vi "Test Autophase.vi"(8 "error in (no error)":errorcluster, 11 "SR7270 Drivers in":refnum<class "SR7270 Drivers.lvclass">) -> (0 "error out":errorcluster, 3 "SR7270 Drivers out":refnum<class "SR7270 Drivers.lvclass">)   [LabVIEW 2016, in "SR7270 Drivers.lvlib"]
uses:
  SR7270 Drivers.lvlib
  <vilib>/addons/_JKI Toolkits/Caraya/classes/Test/Test.lvclass
  Typedefs/REFMODE--enum.ctl
  Typedefs/VRLOCK--enum.ctl
  <vilib>/addons/_JKI Toolkits/Caraya/classes/Assert/Assert.lvclass
  SR7270 Drivers.lvclass
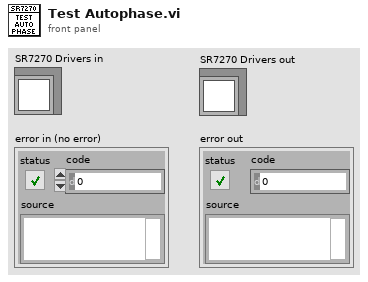
[diagram p1: front panel]
types:
  T1 = typedef "SR7270 Drivers.lvlib/VRLOCK--enum.ctl" = enum16{"Disabled", "Enabled"}
  T2 = typedef "SR7270 Drivers.lvlib/REFMODE--enum.ctl" = enum16{"Single Reference/Virtual Reference", "Dual Harmonic", "Dual Reference"}
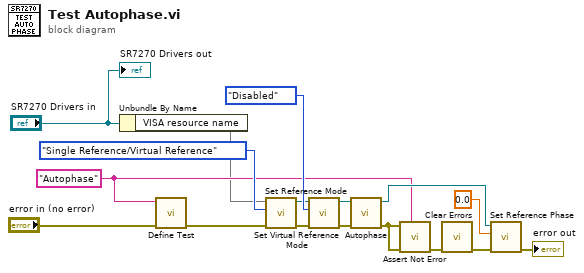
[diagram p0: block diagram]
diagram:
  w3 = "Autophase" ("Label (VI Title)")
  n1 = Unbundle By Name("SR7270 Drivers in") -> ("VISA resource name"=w2)
  n2 = call <vilib>:"Define Test.vi"("error in (no error)"="error in (no error)", "Label (VI Title)"=w3) -> ("error out"=w7:errorcluster)  [unwired: 9 in]
  n3 = call "Set Reference Mode.vi"("error in (no error)"=w7, "Reference Mode"=REFMODE--enum."Single Reference/Virtual Reference", "VISA resource name"=w2) -> ("error out"=w10:errorcluster, "VISA resource name out"=w8:refnum<visa-resource-name>)  [unwired: 7 in]
  n4 = call "Set Virtual Reference Mode.vi"("error in (no error)"=w10, "Virtual Reference Lock"=VRLOCK--enum."Disabled", "VISA resource name"=w8) -> ("error out"=w6:errorcluster, "VISA resource name out"=w5:refnum<visa-resource-name>)  [unwired: 7 in]
  n5 = call "Autophase.vi"("error in (no error)"=w6, "VISA resource name"=w5) -> ("error out"=w4:errorcluster, "VISA resource name out"=w15:refnum<visa-resource-name>)  [unwired: 8 in]
  n6 = call <vilib>:"Assert Not Error.vi"("Label"=w3, "error in (no error)"=w4, "Not Error?"=w4) -> ("error out"=w17:errorcluster)  [unwired: 8 in]
  n7 = call <vilib>:"Clear Errors.vi"("error in (no error)"=w17) -> ("error out"=w13:errorcluster)  [unwired: 5 in, 1 out]
  n8 = call "Set Reference Phase.vi"("error in (no error)"=w13, "Phase (°)"=0.0, "VISA resource name"=w15) -> ("error out"=→"error out":errorcluster)  [unwired: 7 in, 1 out]
  "SR7270 Drivers out" <- "SR7270 Drivers in"
